vi "Generate Async Msg Event.vi"(7 "AdHoc Msg (\"\")":string, 8 "error in (no error)":errorcluster, 9 "vData":variant, 10 "AsyncMsg":T1, 11 "Temp01 in":refnum<class "TELLC_Temp01.lvclass">) -> (0 "error out":errorcluster, 3 "Temp01 out":refnum<class "TELLC_Temp01.lvclass">)   [LabVIEW 2017, in "TELLC_Temp01.lvclass"]
doc: "Developed by Kevin Thompson\nkevin@thompsonengineering.net\n\nCopyright 2018\nThompson Engineering, LLC"
uses:
  TELLC_Temp01.lvclass
  DataTypes/AsynMsg_Temp01--enum.ctl
  Common/DataTypes/TD Async CmdMsg EventData--cluster.ctl
  TELLC_Temp01.lvclass/TELLC_Temp01.ctl
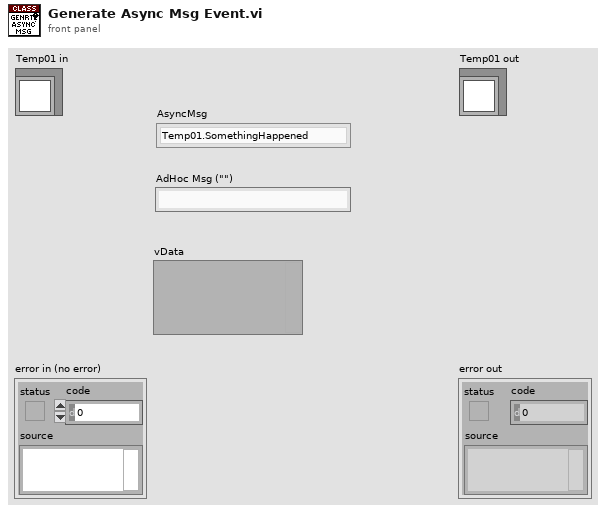
[diagram p1: front panel]
types:
  T1 = typedef "TELLC_Temp01.lvclass/AsynMsg_Temp01--enum.ctl" = enum16{"Temp01.SomethingHappened"}
  T2 = typedef "TD Async CmdMsg EventData--cluster.ctl" = cluster{"Time Stamp":timestamp, "CmdMsg":string, "vData":variant}
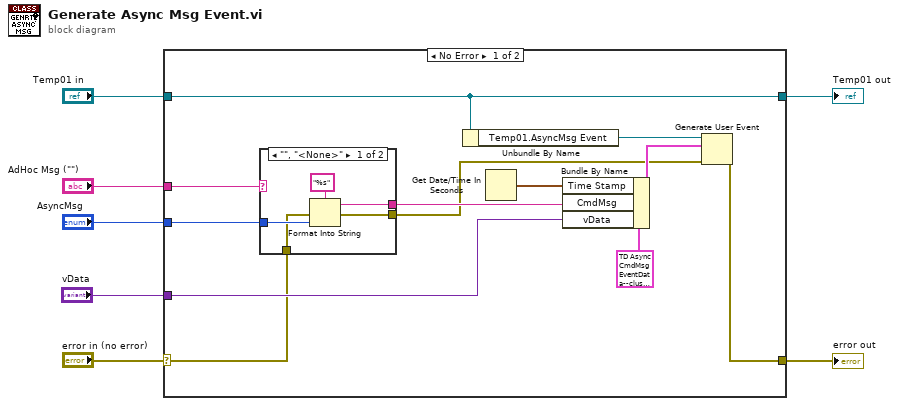
[diagram p0: block diagram]
diagram:
  n1 = case shown="No Error" "error in (no error)" {
    selector: "error in (no error)" -> [w11 w28]
    tunnel: [w18 w28] -> w2
    tunnel: [w12 w27] -> w6
    tunnel: "Temp01 in" -> [w12 w27]
    tunnel: "AsyncMsg" -> [w9 _]
    tunnel: "vData" -> [w13 _]
    tunnel: "AdHoc Msg (\"\")" -> [w8 _]
    frame No Error {
      n2 = case shown="\"\", \"<None>\"" w8 {
        selector: w8 -> [_ w25]
        tunnel: w9 -> [w23 _]
        tunnel: [w22 w25] -> w14
        tunnel: w11 -> [w21 w26]
        tunnel: [w20 w26] -> w10
        frame "", "<None>" {
          n3 = Format Into String(format string="%s", error in=w21, w23) -> (resulting string=w22:string, error out=w20:errorcluster)  [unwired: 1 in]
        }
        frame Default {
        }
      }
      n4 = Unbundle By Name(w12) -> ("Temp01.AsyncMsg Event"=w19:refnum<user-event>)
      n5 = Get Date/Time In Seconds() -> (seconds since 1Jan1904=w15:timestamp)
      n6 = Bundle By Name(cluster=T2 {"Time Stamp"=timestamp(0 s since 1904-01-01), "CmdMsg"="", "vData"=variant} ("Async EvData"), "Time Stamp"=w15, "CmdMsg"=w14, "vData"=w13) -> (w17:T2)
      n7 = Generate User Event(user event=w19, event data cluster=w17, error in=w10) -> (error out=w18:errorcluster)  [unwired: 1 in, 1 out]
    }
    frame Error {
    }
  }
  "error out" <- w2
  "Temp01 out" <- w6
